vi "svfa_Average Array (real) No State.vi"(6 "averaging state info in":T2={"complex FFT"=[], "real FFT"=[], "f0"=0.0, "df"=0.0, "averages completed"=0.0, "averaging parameters"={"averaging mode"=enum."No averaging", "weighting mode"=enum."Linear", "number of averages"=10, "linear mode"=enum."Auto restart"}} {"averages completed" format="%.2f"; "df" format="%.2f"; "f0" format="%.2f"; "real FFT" format="%.2f"; "complex FFT" format="%.2f"}, 7 "processing control":T1(ring), 11 "array":dbl[](array[numeric]) format="%.2f") -> (0 "averages completed":dbl, 1 "averaging done":bool, 3 "average array":dbl[](array[numeric]) format="%.2f", 4 "averaging state info out":T3={"complex FFT"=[], "Mag/Real FFT"=[], "f0"=0.0, "df"=0.0, "averages completed"=0.0, "averaging parameters"={"averaging mode"=enum."No averaging", "weighting mode"=enum."Linear", "number of averages"=10, "linear mode"=enum."Auto restart"}} {"averages completed" format="%.2f"; "df" format="%.2f"; "f0" format="%.2f"; "Mag/Real FFT" format="%.2f"; "complex FFT" format="%.2f"})   [LabVIEW 2017]
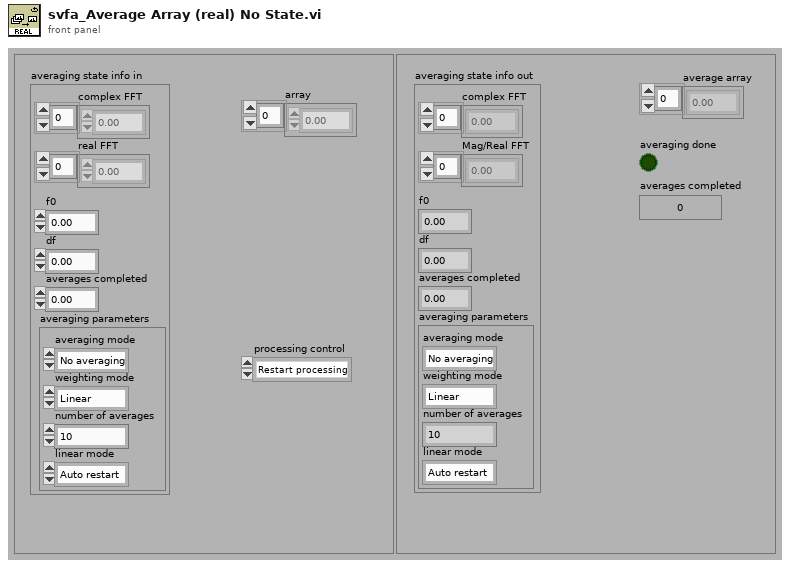
[diagram p1: front panel]
types:
  T1 = enum16{"Restart processing", "Continue processing", "Skip processing"}
  T2 = cluster{"complex FFT":cdb[], "real FFT":dbl[], "f0":dbl, "df":dbl, "averages completed":dbl, "averaging parameters":cluster{"averaging mode":enum16{"No averaging", "Vector averaging", "RMS averaging", "Peak hold"}, "weighting mode":enum16{"Linear", "Exponential"}, "number of averages":u32, "linear mode":enum16{"One shot", "Auto restart"}}}
  T3 = cluster{"complex FFT":cdb[], "Mag/Real FFT":dbl[], "f0":dbl, "df":dbl, "averages completed":dbl, "averaging parameters":cluster{"averaging mode":enum16{"No averaging", "Vector averaging", "RMS averaging", "Peak hold"}, "weighting mode":enum16{"Linear", "Exponential"}, "number of averages":u32, "linear mode":enum16{"One shot", "Auto restart"}}}
  T4 = enum16{"No averaging", "Vector averaging", "RMS averaging", "Peak hold"}
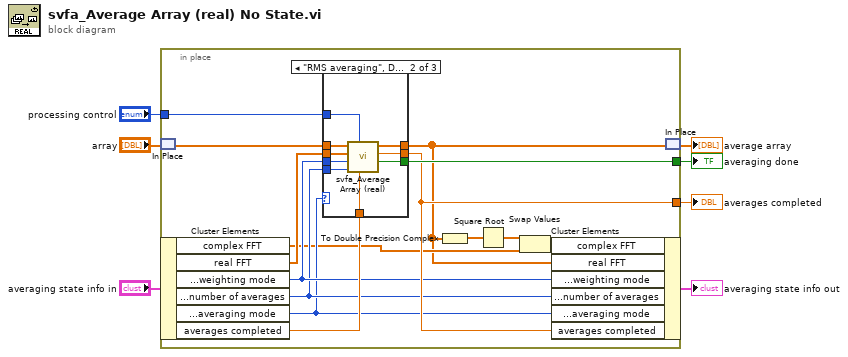
[diagram p0: block diagram]
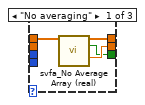
[diagram p2: hidden frame]
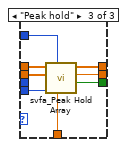
[diagram p3: hidden frame]
diagram:
  n1 = in-place {
    in-place-border: [w17] -> w7
    in-place-border: [w21] -> w6
    in-place-border: "processing control" -> [w20]
    n2 = in-place-match #1("array") -> (w11:dbl[])
    n3 = in-place-cluster #2("averaging state info in") -> ("complex FFT"=w13:cdb[], "real FFT"=w19:dbl[], "averaging parameters.weighting mode"=w16:enum16{"Linear", "Exponential"}, "averaging parameters.number of averages"=w15:u32, "averaging parameters.averaging mode"=w14:T4, "averages completed"=w18:dbl)
    n4 = case shown="\"RMS averaging\", Default" w14 {
      tunnel: [w24 w34 w41] -> w10
      tunnel: [w23 w33 w36] -> w17
      tunnel: w11 -> [w25 w32 w42]
      tunnel: [w22 w31 w35] -> w21
      tunnel: w18 -> [_ w30 w37]
      tunnel: w16 -> [_ w29 _]
      tunnel: w19 -> [_ w28 w39]
      tunnel: w15 -> [_ w27 w38]
      tunnel: w20 -> [_ w26 w40]
      frame "No averaging" {
        n5 = call <vilib>:"svfa_No Average Array (real).vi"("spectrum"=w25) -> ("dup spectrum"=w24:dbl[], "new spectrum ready"=w22:bool, "averages completed"=w23:dbl)  [unwired: 10 in, 2 out]
      }
      frame "RMS averaging", Default {
        n6 = call <vilib>:"svfa_Average Array (real).vi"("averages completed in"=w30, "processing control"=w26, "number of averages"=w27, "weighting mode"=w29, "previous average array"=w28, "array"=w32) -> ("averaging done"=w31:bool, "averages completed out"=w33:dbl, "average array"=w34:dbl[])  [unwired: 3 in]
      }
      frame "Peak hold" {
        n7 = call <vilib>:"svfa_Peak Hold Array.vi"("averages completed in"=w37, "processing control"=w40, "number of averages"=w38, "previous peak array"=w39, "array"=w42) -> ("averaging done"=w35:bool, "averages completed out"=w36:dbl, "peak array"=w41:dbl[])  [unwired: 4 in]
      }
    }
    n8 = To Double Precision Complex(1:w10) -> (0:w9:cdb[])
    n9 = Square Root(x=w9) -> (sqrt(x)=w8:cdb[])
    n10 = Swap Values(12:w8, 14:w13) -> (3:w12:cdb[])  [unwired: 1 in, 1 out]
    n11 = in-place-cluster #2("complex FFT"=w12, "real FFT"=w10, "averaging parameters.weighting mode"=w16, "averaging parameters.number of averages"=w15, "averaging parameters.averaging mode"=w14, "averages completed"=w17) -> (→"averaging state info out":T2)
    n12 = in-place-match #1(w10) -> (→"average array":dbl[])
  }
  "averages completed" <- w7
  "averaging done" <- w6
